vi "MAC to Label.vi"(8 "Error In":errorcluster, 11 "MAC address":string) -> (0 "Error Out":errorcluster, 3 "Label":string)   [LabVIEW 2016]
uses:
  <vilib>/Utility/file.llb/Read Delimited Spreadsheet (string).vi
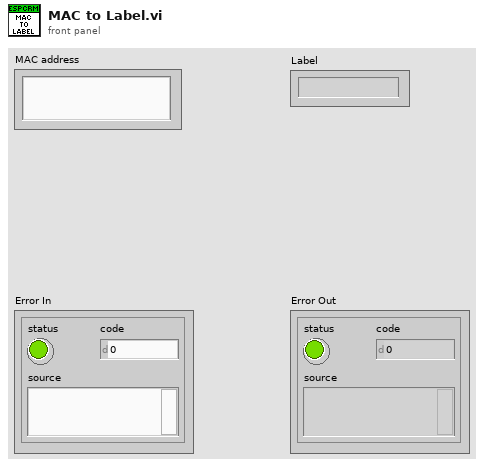
[diagram p1: front panel]
types:
  T1 = enum16{"open", "replace", "create", "open or create", "replace or create", "replace or create with confirmation"}
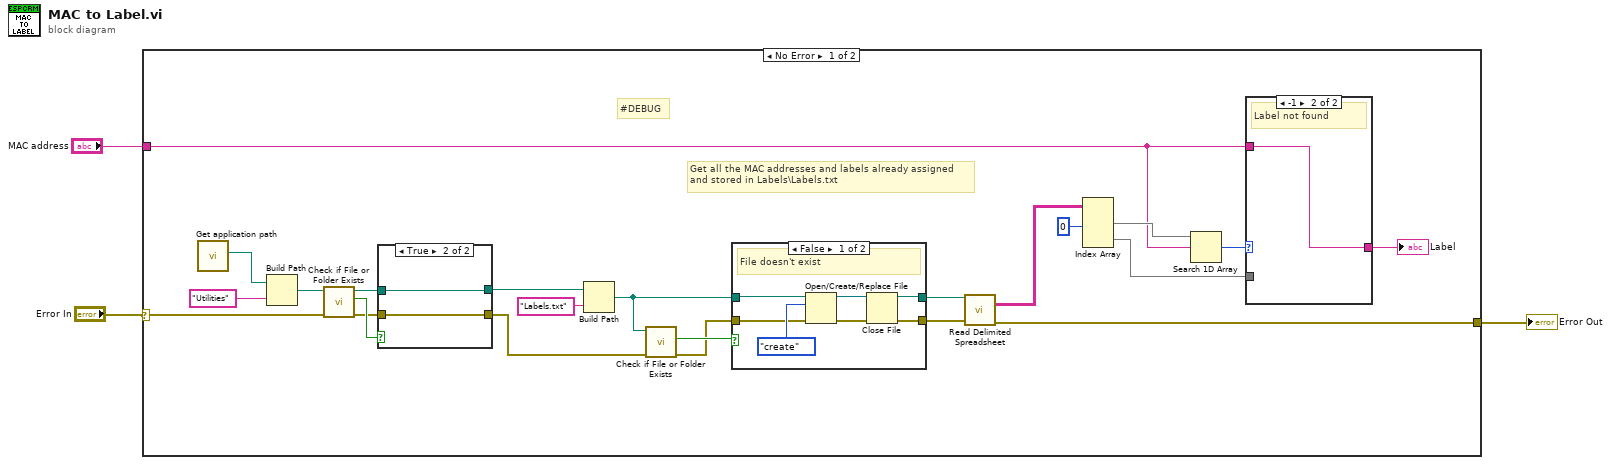
[diagram p0: block diagram]
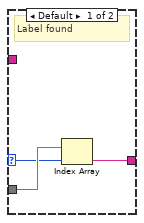
[diagram p2: hidden frame]
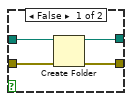
[diagram p3: hidden frame]
diagram:
  n1 = case shown="No Error" "Error In" {
    selector: "Error In" -> [w5 w46]
    tunnel: [w10 w46] -> w3
    tunnel: "MAC address" -> [w4 _]
    frame No Error {
      # "#DEBUG"
      # "Get all the MAC addresses and labels already assigned\nand stored in Labels\\Labels.txt"
      n2 = call "Get application path.vi"() -> ("Application path"=w14:path)  [unwired: 11 in]
      n3 = Build Path(base path=w14, name or relative path="Utilities") -> (appended path=w16:path)
      n4 = call <vilib>:"Check if File or Folder Exists.vi"("error in (no error)"=w5, "path"=w16) -> ("error out"=w20:errorcluster, "file or folder exists?"=w21:bool, "dup path"=w19:path)  [unwired: 7 in]
      n5 = case shown="True" w21 {
        tunnel: w20 -> [w34 w35]
        tunnel: w19 -> [w33 w36]
        tunnel: [w32 w36] -> w18
        tunnel: [w31 w35] -> w13
        frame False {
          n6 = Create Folder(path (use dialog)=w33, error in=w34) -> (created path=w32:path, error out=w31:errorcluster)  [unwired: 1 in, 1 out]
        }
        frame True {
        }
      }
      n7 = Build Path(base path=w18, name or relative path="Labels.txt") -> (appended path=w22:path)
      n8 = call <vilib>:"Check if File or Folder Exists.vi"("error in (no error)"=w13, "path"=w22) -> ("error out"=w12:errorcluster, "file or folder exists?"=w23:bool)  [unwired: 7 in, 1 out]
      n9 = case shown="False" w23 {
        tunnel: [w40 w45] -> w24
        tunnel: w22 -> [w39 w45]
        tunnel: w12 -> [w38 w44]
        tunnel: [w37 w44] -> w11
        frame False {
          # "File doesn't exist"
          n10 = Open/Create/Replace File(file path (use dialog)=w39, error in=w38, operation (0:open)=T1."create") -> (refnum out=w41:refnum<file>, error out=w42:errorcluster)  [unwired: 3 in, 1 out]
          n11 = Close File(refnum=w41, error in=w42) -> (path=w40:path, error out=w37:errorcluster)
        }
        frame True {
          # "File exist"
        }
      }
      n12 = call-poly <vilib>:"Read Delimited Spreadsheet.vi"("file path (dialog if empty)"=w24, "error in (no error)"=w11) -> ("all rows"=w26:string[][], "error out"=w10:errorcluster)  [unwired: 8 in, 4 out]
      n13 = Index Array(array=w26, index (col) #1=0 ("disabled index (col)")) -> (element #1=w9:string[], element #2=w7:string[])  [unwired: 3 in]
      n14 = Search 1D Array(1D array=w9, element=w4) -> (index of element=w8:i32)  [unwired: 1 in]
      n15 = case shown="-1" w8 {
        selector: w8 -> [w28 _]
        tunnel: w7 -> [w29 _]
        tunnel: [w27 w30] -> w6
        tunnel: w4 -> [_ w30]
        frame Default {
          # "Label found"
          n16 = Index Array(array=w29, index=w28) -> (element=w27:string)
        }
        frame -1 {
          # "Label not found"
        }
      }
      "Label" <- w6
    }
    frame Error {
    }
  }
  "Error Out" <- w3
